vi "201_SetGetSingle.vi"() -> ()   [LabVIEW 2009]
uses:
  <instrlib>/Zurich Instruments LabOne/Public/Configure/ziGetValueDouble.vi
  <instrlib>/Zurich Instruments LabOne/Public/Configure/ziSetValueDouble.vi
  <instrlib>/Zurich Instruments LabOne/Zurich Instruments LabOne.lvlib
panel:
  out "Set node":string="sigouts/0/on"
  out "Connected?":bool
  out "Value Get":dbl
  out "Error Out":errorcluster
  in  "Address":string="DEV"
  # "Set and Get a single parameter\nThis VI shows how to configure your instrument by assigning a value to a defined data server node. The default node is signout/0/on, which turns on the signal output of the instrument. \n\nSee block diagram for the VI description\n\nRequirements: Any Zurich Instrument Product\n\nTo run\n1- Type the Instrument ID \n2- Run the VI. It will turn on the signal output of the instrument.\n* You can change Node1 and Value1 Set in the back panel to set different nodes \n\nTested Devices:\n- HF2LI\n- UHFLI\n- MFLI\n\n(c) Zurich Instruments.  ALL RIGHTS RESERVED."
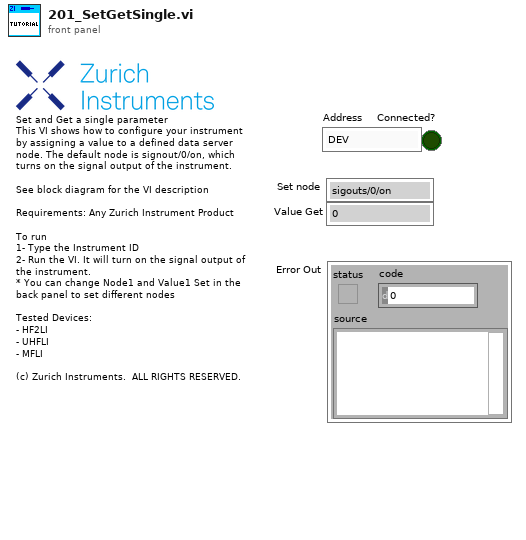
[diagram p1: front panel]
types:
  T1 = typedef "Zurich Instruments LabOne.lvlib/ziTypeHandle.ctl" = cluster{"handleValid":bool, "Conn":u64, "Path Prefix":string, "Handle":u64, "Connected":bool, "Clockbase(s)":dbl}
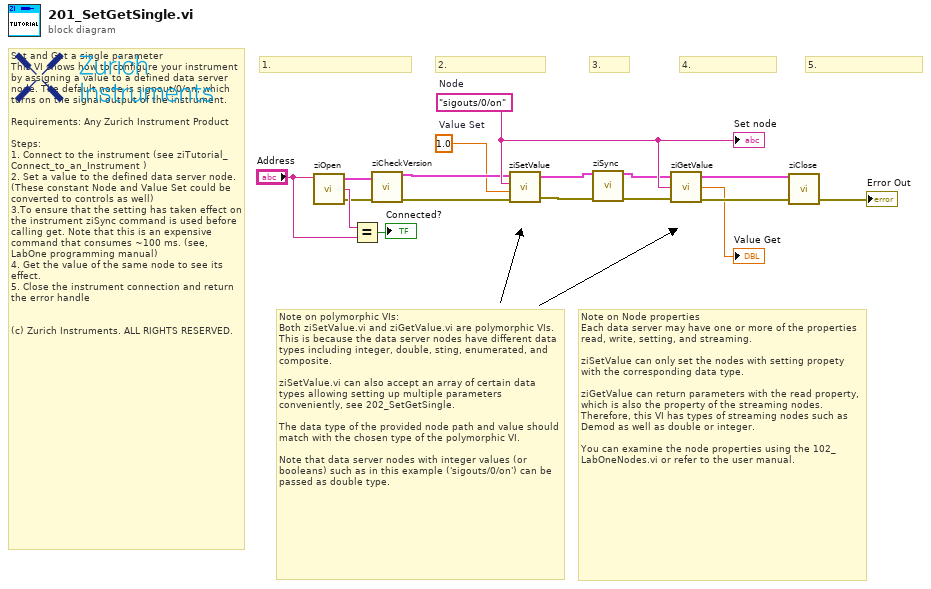
[diagram p0: block diagram]
diagram:
  w1 = 1.0  # Value Set
  w16 = "sigouts/0/on"  # Node
  # "Note on Node properties\nEach data server may have one or more of the properties read, write, setting, and streaming. \n\nziSetValue can only set the nodes with setting propety with the corresponding data type. \n\nziGetValue can return parameters with the read property, which is also the property of the streaming nodes. Therefore, this VI has types of streaming nodes such as Demod as well as double or integer.\n\nYou can examine the node properties using the 102_LabOneNodes.vi or refer to the user manual."
  # "Note on polymorphic VIs:\nBoth ziSetValue.vi and ziGetValue.vi are polymorphic VIs. This is because the data server nodes have different data types including integer, double, sting, enumerated, and composite. \n\nziSetValue.vi can also accept an array of certain data types allowing setting up multiple parameters conveniently, see 202_SetGetSingle. \n\nThe data type of the provided node path and value should match with the chosen type of the polymorphic VI. \n\nNote that data server nodes with integer values (or booleans) such as in this example ('sigouts/0/on') can be passed as double type."
  # "4."
  # "3."
  # "2."
  # "1."
  # "5."
  # "Set and Get a single parameter\nThis VI shows how to configure your instrument by assigning a value to a defined data server node. The default node is signout/0/on, which turns on the signal output of the instrument. \n\nRequirements: Any Zurich Instrument Product\n\nSteps:\n1. Connect to the instrument (see ziTutorial_Connect_to_an_Instrument )\n2. Set a value to the defined data server node. (These constant Node and Value Set could be converted to controls as well) \n3.To ensure that the setting has taken effect on the instrument ziSync command is used before calling get. Note that this is an expensive command that consumes ~100 ms. (see, LabOne programming manual)\n4. Get the value of the same node to see its effect.  \n5. Close the instrument connection and return the error handle   \n\n\n(c) Zurich Instruments. ALL RIGHTS RESERVED."
  n1 = call <instrlib>:"ziOpen.vi"("Address"="Address") -> ("Error Out"=w2:errorcluster, "Selected Device"=w6:string, "HandleOut"=w4:T1)  [unwired: 1 in, 2 out]
  n2 = Equal?(x=w6, y="Address") -> (x = y?=→"Connected?":bool)
  n3 = call <instrlib>:"ziCheckVersion.vi"("Handle In"=w4, "Error In"=w2) -> ("Handle Out"=w8:T1, "Error Out"=w3:errorcluster)  [unwired: 11 in, 1 out]
  n4 = call-poly <instrlib>:"ziSetValue.vi"("Error In"=w3, "Value"=w1, "Path"=w16, "Handle In"=w8) -> ("Error Out"=w12:errorcluster, "Handle Out"=w10:T1)  [unwired: 1 in]
  n5 = call <instrlib>:"ziSync.vi"("Handle In"=w10, "Error In"=w12) -> ("Handle Out"=w9:T1, "Error Out"=w11:errorcluster)  [unwired: 12 in]
  n6 = call-poly <instrlib>:"ziGetValue.vi"("error in"=w11, "Path"=w16, "Handle in"=w9) -> ("error out"=w14:errorcluster, "Value"=→"Value Get":dbl, "Handle out"=w15:T1)
  n7 = call <instrlib>:"ziClose.vi"("Error In"=w14, "Handle In"=w15) -> ("Error Out"=→"Error Out":errorcluster)  [unwired: 2 in, 1 out]
  "Set node" <- w16
